vi "3ptmed.vi"(1 "s2":fxp<+/-,24,5>, 2 "s1":fxp<+/-,24,5>, 3 "s0":fxp<+/-,24,5>) -> (0 "sout":fxp<+/-,24,5> format="%.21g")   [LabVIEW 2013]
doc: "Find the median of three input values"
uses:
  <vilib>/rvi/Emulation/niFpgaSctlEmulationGetInTimedLoop.vi
  <vilib>/rvi/Emulation/niFpgaProcessEmulError.vi
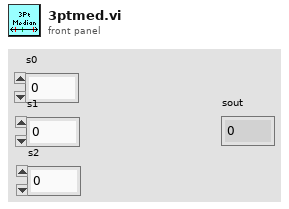
[diagram p1: front panel]
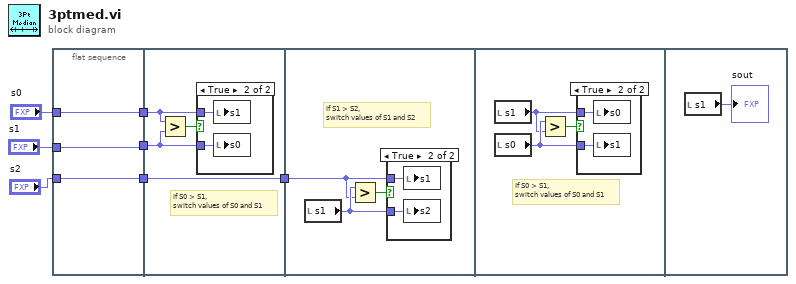
[diagram p0: block diagram]
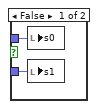
[diagram p2: hidden frame]
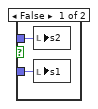
[diagram p3: hidden frame]
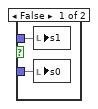
[diagram p4: hidden frame]
diagram:
  n1 = flat-sequence {
    tunnel: "s0" -> [w10]
    tunnel: [w10] -> w5
    tunnel: [w8] -> w4
    tunnel: [w9] -> w3
    tunnel: "s2" -> [w9]
    tunnel: "s1" -> [w8]
    tunnel: [w11] -> w7
    tunnel: w5 -> [w13]
    tunnel: w4 -> [w12]
    tunnel: w3 -> [w11]
    tunnel: w7 -> [w19]
    frame #0 {
    }
    frame #1 {
      # "If S0 > S1, \nswitch values of S0 and S1"
      n2 = Greater?(x=w13, y=w12) -> (0:w14:bool)
      n3 = case shown="True" w14 {
        tunnel: w13 -> [w16 w18]
        tunnel: w12 -> [w15 w17]
        frame False {
          n4 = local write "s0"(w16) -> ()
          n5 = local write "s1"(w15) -> ()
        }
        frame True {
          n6 = local write "s1"(w18) -> ()
          n7 = local write "s0"(w17) -> ()
        }
      }
    }
    frame #2 {
      # "If S1 > S2, \nswitch values of S1 and S2"
      n8 = local read "s1"() -> (w20:fxp<+/-,24,5>)
      n9 = Greater?(x=w20, y=w19) -> (0:w21:bool)
      n10 = case shown="True" w21 {
        tunnel: w20 -> [w23 w24]
        tunnel: w19 -> [w22 w25]
        frame False {
          n11 = local write "s2"(w22) -> ()
          n12 = local write "s1"(w23) -> ()
        }
        frame True {
          n13 = local write "s1"(w25) -> ()
          n14 = local write "s2"(w24) -> ()
        }
      }
    }
    frame #3 {
      # "If S0 > S1,\nswitch values of S0 and S1"
      n15 = local read "s1"() -> (w26:fxp<+/-,24,5>)
      n16 = local read "s0"() -> (w27:fxp<+/-,24,5>)
      n17 = Greater?(x=w27, y=w26) -> (0:w28:bool)
      n18 = case shown="True" w28 {
        tunnel: w27 -> [w30 w32]
        tunnel: w26 -> [w29 w31]
        frame False {
          n19 = local write "s1"(w29) -> ()
          n20 = local write "s0"(w30) -> ()
        }
        frame True {
          n21 = local write "s0"(w31) -> ()
          n22 = local write "s1"(w32) -> ()
        }
      }
    }
    frame #4 {
      n23 = local read "s1"() -> (→"sout":fxp<+/-,24,5>)
    }
  }
